vi "Report data in.vi"(11 "Cluster 2":T2) -> (3 "output cluster 4":T1)   [LabVIEW 2015]
uses:
  Galobal variable_TI.vi
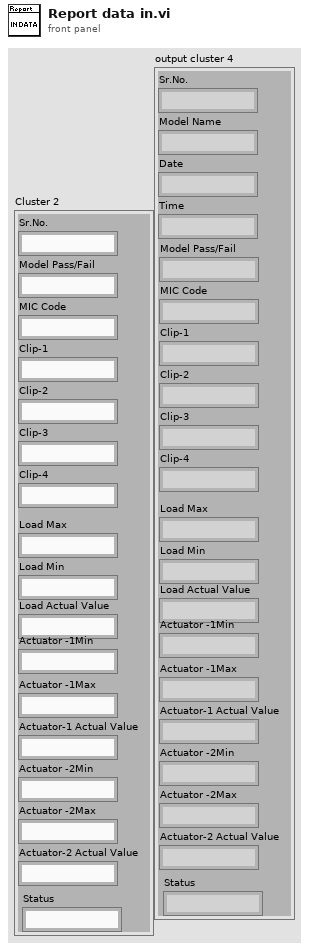
[diagram p1: front panel]
types:
  T1 = cluster{"Sr.No.":string, "Model Name":string, "Date":string, "Time":string, "Model Pass/Fail":string, "MIC Code":string, "Clip-1":string, "Clip-2":string, "Clip-3":string, "Clip-4":string, "Load Max":string, "Load Min":string, "Load Actual Value":string, "Actuator -1Min":string, "Actuator -1Max":string, "Actuator-1 Actual Value":string, "Actuator -2Min ":string, "Actuator -2Max ":string, "Actuator-2 Actual Value ":string, "Status":string}
  T2 = cluster{"Sr.No.":string, "Model Pass/Fail":string, "MIC Code":string, "Clip-1":string, "Clip-2":string, "Clip-3":string, "Clip-4":string, "Load Max":string, "Load Min":string, "Load Actual Value":string, "Actuator -1Min":string, "Actuator -1Max":string, "Actuator-1 Actual Value":string, "Actuator -2Min ":string, "Actuator -2Max ":string, "Actuator-2 Actual Value ":string, "Status":string}
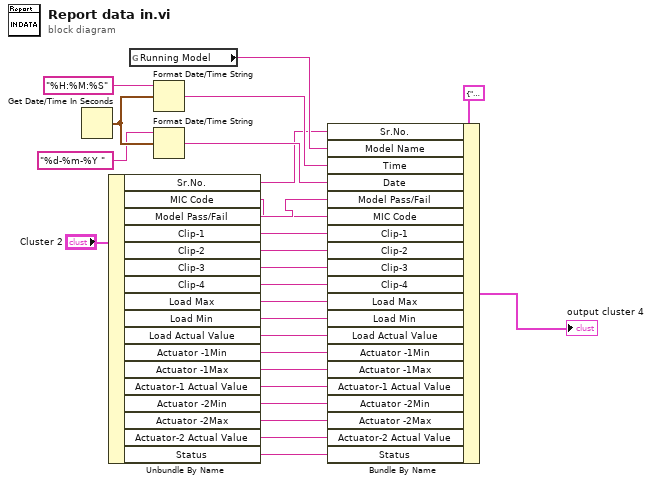
[diagram p0: block diagram]
diagram:
  n1 = Get Date/Time In Seconds() -> (seconds since 1Jan1904=w23:timestamp)
  n2 = Unbundle By Name("Cluster 2") -> ("Sr.No."=w20:string, "MIC Code"=w15:string, "Model Pass/Fail"=w16:string, "Clip-1"=w14:string, "Clip-2"=w13:string, "Clip-3"=w12:string, "Clip-4"=w11:string, "Load Max"=w10:string, "Load Min"=w9:string, "Load Actual Value"=w8:string, "Actuator -1Min"=w7:string, "Actuator -1Max"=w6:string, "Actuator-1 Actual Value"=w5:string, "Actuator -2Min"=w4:string, "Actuator -2Max"=w3:string, "Actuator-2 Actual Value"=w2:string, "Status"=w1:string)
  n3 = global read "Galobal variable_TI.vi" "Running Model"() -> (w26:string)
  n4 = Format Date/Time String(time format string (%c)="%H:%M:%S", seconds (now)=w23) -> (date/time string=w24:string)  [unwired: 1 in]
  n5 = Format Date/Time String(time format string (%c)="%d-%m-%Y ", seconds (now)=w23) -> (date/time string=w25:string)  [unwired: 1 in]
  n6 = Bundle By Name(cluster=T1 {"Sr.No."="", "Model Name"="", "Date"="", "Time"="", "Model Pass/Fail"="", "MIC Code"="", "Clip-1"="", "Clip-2"="", "Clip-3"="", "Clip-4"="", "Load Max"="", "Load Min"="", "Load Actual Value"="", "Actuator -1Min"="", "Actuator -1Max"="", "Actuator-1 Actual Value"="", "Actuator -2Min "="", "Actuator -2Max "="", "Actuator-2 Actual Value "="", "Status"=""} ("output cluster 2"), "Sr.No."=w20, "Model Name"=w26, "Time"=w24, "Date"=w25, "Model Pass/Fail"=w16, "MIC Code"=w15, "Clip-1"=w14, "Clip-2"=w13, "Clip-3"=w12, "Clip-4"=w11, "Load Max"=w10, "Load Min"=w9, "Load Actual Value"=w8, "Actuator -1Min"=w7, "Actuator -1Max"=w6, "Actuator-1 Actual Value"=w5, "Actuator -2Min"=w4, "Actuator -2Max"=w3, "Actuator-2 Actual Value"=w2, "Status"=w1) -> (→"output cluster 4":T1)
